vi "Get Waveform In Range.vi"(7 "Ignore Wfm Timestamps?":bool, 8 "error in (no error)":errorcluster, 9 "Data in":dbl[](array[numeric]), 10 "Current Wfm":T6, 11 "Log Instance in":T1) -> (0 "error out":errorcluster, 1 "Data out":dbl[](array[numeric]), 2 "Waveform Data":T5, 3 "Log Instance out":T1, 4 "tf Modified?":bool, 5 "In Range?":bool)   [LabVIEW 2012, in "Waveform Data Logger Engine.lvlib" / "Waveform Log.lvclass"]
uses:
  Waveform Log.lvclass
  Log Instance.ctl
  Logs/Segmented Logs/Segmented Log/Segmented Log.lvclass
  Log Instance Waveform.ctl
  Waveform Information.ctl
  Waveform Data Type.ctl
  Waveform Receive/Wfm Info.ctl
  Waveform Log Wfm Meta Data.ctl
  Waveform Receive/Waveform Receive.lvclass
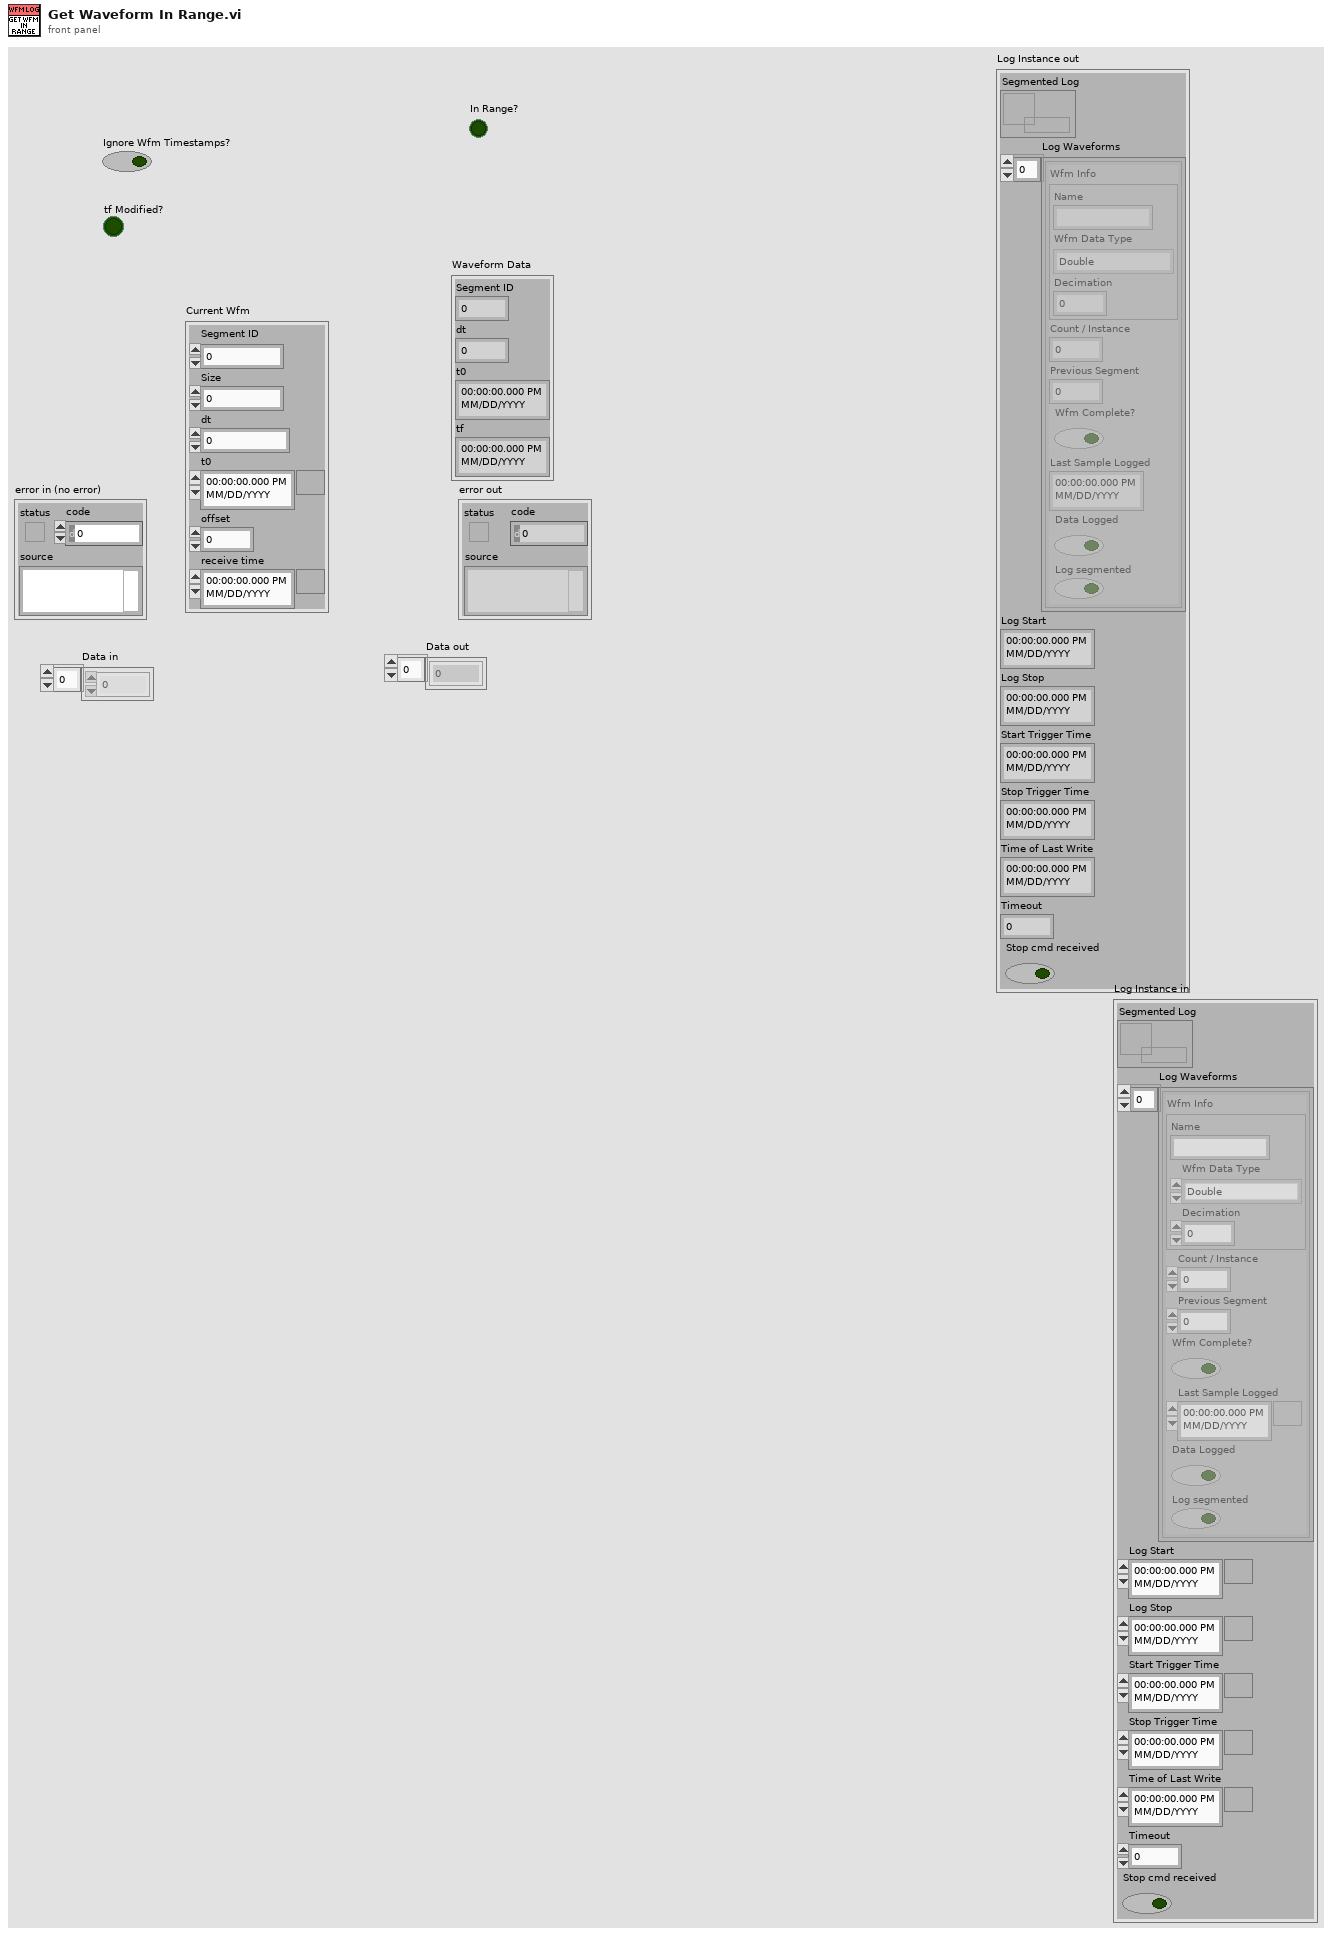
[diagram p1: front panel]
types:
  T1 = typedef "Waveform Data Logger Engine.lvlib/Waveform Log.lvclass/Log Instance.ctl" = cluster{"Segmented Log":refnum<data-value>, "Log Waveforms":T2[], "Log Start":timestamp, "Log Stop":timestamp, "Start Trigger Time":timestamp, "Stop Trigger Time":timestamp, "Time of Last Write":timestamp, "Timeout":dbl, "Stop cmd received":bool}
  T2 = typedef "Waveform Data Logger Engine.lvlib/Waveform Log.lvclass/Log Instance Waveform.ctl" = cluster{"Wfm Info":T3, "Count / Instance":i32, "Previous Segment":u64, "Wfm Complete?":bool, "Last Sample Logged":timestamp, "Data Logged":bool, "Log segmented":bool}
  T3 = typedef "Waveform Data Logger Engine.lvlib/Waveform Log.lvclass/Waveform Information.ctl" = cluster{"Name":string, "Wfm Data Type":T4, "Decimation":u32}
  T4 = typedef "Waveform Data Logger Engine.lvlib/Waveform Log.lvclass/Waveform Data Type.ctl" = enum16{"Double", "ComplexDouble"}
  T5 = typedef "Waveform Data Logger Engine.lvlib/Waveform Log.lvclass/Waveform Log Wfm Meta Data.ctl" = cluster{"Segment ID":u64, "dt":dbl, "t0":timestamp, "tf":timestamp}
  T6 = typedef "Waveform Data Logger Engine.lvlib/Waveform Receive.lvclass/Wfm Info.ctl" = cluster{"Segment ID":u64, "Size":i32, "dt":dbl, "t0":timestamp, "offset":u64, "receive time":timestamp}
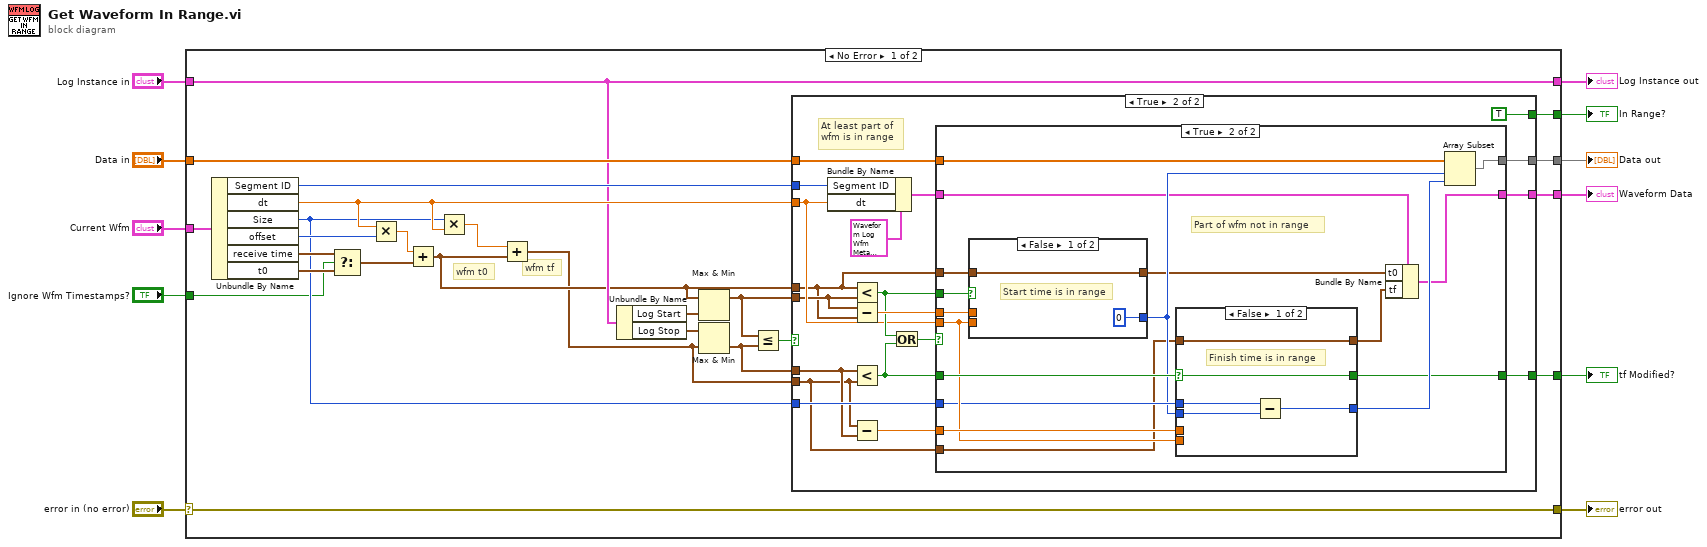
[diagram p0: block diagram]
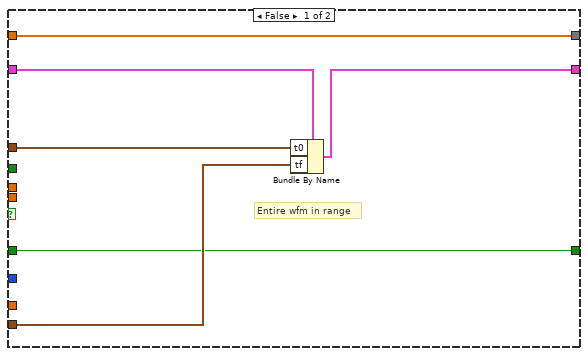
[diagram p3: hidden frame]
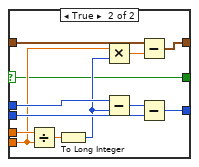
[diagram p4: hidden frame]
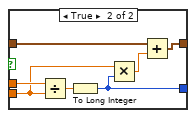
[diagram p5: hidden frame]
diagram:
  n1 = case shown="No Error" "error in (no error)" {
    selector: "error in (no error)" -> [w36 w108]
    tunnel: [w36 w108] -> w10
    tunnel: [w16 w106] -> w9
    tunnel: "Current Wfm" -> [w24 _]
    tunnel: [w23 _] -> w7
    tunnel: "Data in" -> [w22 w107]
    tunnel: [w21 w107] -> w5
    tunnel: [w17 _] -> w4
    tunnel: "Log Instance in" -> [w16 w106]
    tunnel: "Ignore Wfm Timestamps?" -> [w15 _]
    tunnel: [w12 _] -> w1
    frame No Error {
      # "wfm tf"
      # "wfm t0"
      n2 = Unbundle By Name(w24) -> ("Segment ID"=w19:u64, "dt"=w20:dbl, "Size"=w18:i32, "offset"=w30:u64, "receive time"=w31:timestamp, "t0"=w32:timestamp)
      n3 = Select(t=w31, s=w15, f=w32) -> (s? t:f=w33:timestamp)
      n4 = Multiply(x=w20, y=w30) -> (x*y=w34:dbl)
      n5 = Add(x=w34, y=w33) -> (x+y=w14:timestamp)
      n6 = Multiply(x=w18, y=w20) -> (x*y=w35:dbl)
      n7 = Add(x=w35, y=w14) -> (x+y=w13:timestamp)
      n8 = Unbundle By Name(w16) -> ("Log Start"=w29:timestamp, "Log Stop"=w28:timestamp)
      n9 = Max & Min(x=w14, y=w29) -> (max(x,y)=w26:timestamp)  [unwired: 1 out]
      n10 = Max & Min(x=w28, y=w13) -> (min(x,y)=w25:timestamp)  [unwired: 1 out]
      n11 = Less Or Equal?(x=w26, y=w25) -> (x <= y?=w27:bool)
      n12 = case shown="True" w27 {
        tunnel: w26 -> [_ w44]
        tunnel: w25 -> [_ w43]
        tunnel: w13 -> [_ w39]
        tunnel: w14 -> [_ w40]
        tunnel: [_ TRUE] -> w23
        tunnel: w22 -> [w37 w54]
        tunnel: [w37 w49] -> w21
        tunnel: w20 -> [_ w46]
        tunnel: w18 -> [_ w51]
        tunnel: w19 -> [_ w47]
        tunnel: [_ w41] -> w17
        tunnel: [_ w38] -> w12
        frame False {
          # "Wfm not in range"
        }
        frame True {
          # "At least part of \nwfm is in range"
          n13 = Bundle By Name(cluster=T5 {"Segment ID"=0, "dt"=0.0, "t0"=timestamp(0 s since 1904-01-01), "tf"=timestamp(0 s since 1904-01-01)} ("Waveform Data"), "Segment ID"=w47, "dt"=w46) -> (w42:T5)
          n14 = Less?(x=w40, y=w44) -> (x < y?=w52:bool)
          n15 = Subtract(x=w44, y=w40) -> (x-y=w56:dbl)
          n16 = Less?(x=w43, y=w39) -> (x < y?=w53:bool)
          n17 = Subtract(x=w39, y=w43) -> (x-y=w55:dbl)
          n18 = Or(x=w52, y=w53) -> (x .or. y?=w50:bool)
          n19 = case shown="True" w50 {
            tunnel: w56 -> [_ w79]
            tunnel: w55 -> [_ w78]
            tunnel: w54 -> [w62 w77]
            tunnel: w53 -> [w57 w76]
            tunnel: w52 -> [_ w75]
            tunnel: w46 -> [_ w74]
            tunnel: w51 -> [_ w73]
            tunnel: [w62 w70] -> w49
            tunnel: w40 -> [w61 w69]
            tunnel: w39 -> [w60 w67]
            tunnel: w42 -> [w59 w65]
            tunnel: [w58 w64] -> w41
            tunnel: [w57 w63] -> w38
            frame False {
              # "Entire wfm in range"
              n20 = Bundle By Name(cluster=w59, "t0"=w61, "tf"=w60) -> (w58:T5)
            }
            frame True {
              # "Part of wfm not in range"
              n21 = case shown="False" w75 {
                tunnel: w79 -> [_ w104]
                tunnel: w74 -> [_ w103]
                tunnel: [0 w102] -> w72
                tunnel: w69 -> [w97 w99]
                tunnel: [w97 w101] -> w68
                frame False {
                  # "Start time is in range"
                }
                frame True {
                  n22 = Divide(x=w104, y=w103) -> (x/y=w105:dbl)
                  n23 = To Long Integer(number=w105) -> (32bit integer=w102:i32)
                  n24 = Multiply(x=w103, y=w102) -> (x*y=w100:dbl)
                  n25 = Add(x=w99, y=w100) -> (x+y=w101:timestamp)
                }
              }
              n26 = case shown="False" w76 {
                selector: w76 -> [w80 w85]
                tunnel: w78 -> [_ w95]
                tunnel: w74 -> [_ w90]
                tunnel: w73 -> [w84 w94]
                tunnel: w72 -> [w83 w92]
                tunnel: [w82 w91] -> w71
                tunnel: w67 -> [w81 w88]
                tunnel: [w81 w86] -> w66
                tunnel: [w80 w85] -> w63
                frame False {
                  # "Finish time is in range"
                  n27 = Subtract(x=w84, y=w83) -> (x-y=w82:i32)
                }
                frame True {
                  n28 = Divide(x=w95, y=w90) -> (x/y=w96:dbl)
                  n29 = To Long Integer(number=w96) -> (32bit integer=w89:i32)
                  n30 = Multiply(x=w90, y=w89) -> (x*y=w87:dbl)
                  n31 = Subtract(x=w94, y=w89) -> (x-y=w93:i32)
                  n32 = Subtract(x=w88, y=w87) -> (x-y=w86:timestamp)
                  n33 = Subtract(x=w93, y=w92) -> (x-y=w91:i32)
                }
              }
              n34 = Bundle By Name(cluster=w65, "t0"=w68, "tf"=w66) -> (w64:T5)
              n35 = Array Subset(array=w77, index=w72, length=w71) -> (w70:dbl[])
            }
          }
        }
      }
    }
    frame Error {
    }
  }
  "error out" <- w10
  "Log Instance out" <- w9
  "Waveform Data" <- w4
  "Data out" <- w5
  "In Range?" <- w7
  "tf Modified?" <- w1
